vi "Pcre2JitCompile8.vi"(8 "error in":errorcluster, 9 "Options (1)":u32=1 format="%.0x", 11 "pCode":u64 format="%.0x") -> (0 "error out":errorcluster, 3 "pCode":u64 format="%.0x")   [LabVIEW 2021, in "libpcre2-8.lvlib"]
uses:
  libpcre2-8.lvlib
  libpcre2-8-x32.dll
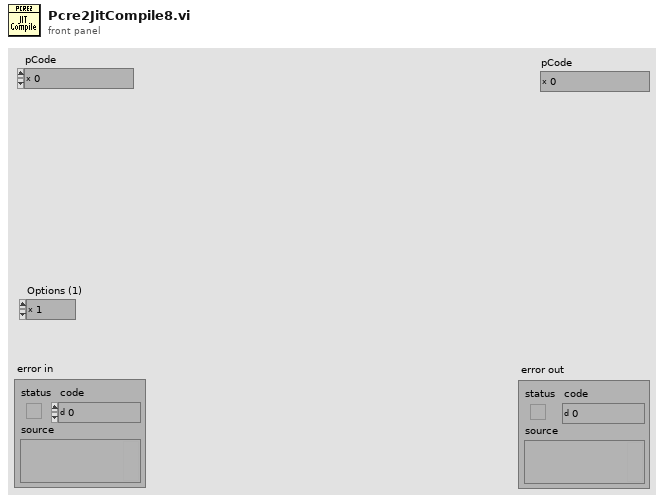
[diagram p1: front panel]
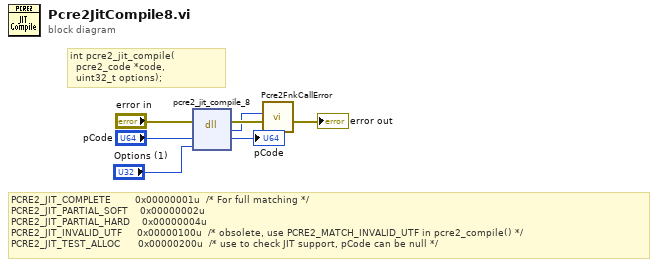
[diagram p0: block diagram]
diagram:
  # "PCRE2_JIT_COMPLETE        0x00000001u  /* For full matching */\nPCRE2_JIT_PARTIAL_SOFT    0x00000002u\nPCRE2_JIT_PARTIAL_HARD    0x00000004u\nPCRE2_JIT_INVALID_UTF     0x00000100u  /* obsolete, use PCRE2_MATCH_INVALID_UTF in pcre2_compile() */\nPCRE2_JIT_TEST_ALLOC      0x00000200u  /* use to check JIT support, pCode can be null */"
  # "int pcre2_jit_compile(\n  pcre2_code *code, \n  uint32_t options);"
  n1 = dll-call lib="libpcre2-8-x*.dll" fn="pcre2_jit_compile_8"(error in="error in", "code"="pCode", "options"="Options (1)") -> (error out=w3:errorcluster, "return"=w1:i32, "code"=→"pCode":u64)  [unwired: 3 in, 1 out]
  n2 = call "Pcre2FnkCallError.vi"("error in"=w3, "ErrorCode"=w1) -> ("error out"=→"error out":errorcluster)  [unwired: 9 in]
